vi "Clear Str Space.vi"(11 "SN":string) -> (3 "字符串":string)   [LabVIEW 2014]
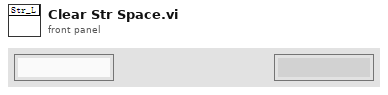
[diagram p1: front panel]
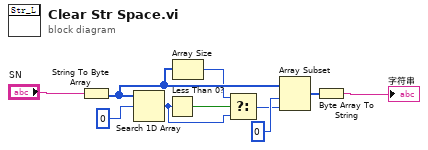
[diagram p0: block diagram]
diagram:
  n1 = String To Byte Array(string="SN") -> (unsigned byte array=w5:u8[])
  n2 = Search 1D Array(1D array=w5, element=u8 0 ("元素")) -> (index of element=w3:i32)  [unwired: 1 in]
  n3 = Less Than 0?(x=w3) -> (x < 0?=w7:bool)
  n4 = Array Size(array=w5) -> (size(s)=w4:i32)
  n5 = Select(t=w4, s=w7, f=w3) -> (s? t:f=w6:i32)
  n6 = Array Subset(array=w5, index=0 ("索引"), length=w6) -> (w8:u8[])
  n7 = Byte Array To String(unsigned byte array=w8) -> (string=→"字符串":string)
